vi "FPGA_Global.vi"() -> ()   [LabVIEW 2011]
panel:
  in  "Number of Modulation Points":u8
  in  "Cycles per Modulation":u32
  in  "Saturated Position Step":i32
  in  "Mobility Update?":bool
  in  "Cycles per Square Wave":u16
  in  "Square Voltage (y)":i16
  in  "Square Voltage (x)":i16
  in  "Inverse Mobility":i32
  in  "Inverse Diffusion Constant":u32
  in  "Sub-Bin Delay (ticks)":u16
  in  "Bins per Cycle":u8
  in  "Bin Period (ticks)":u16
  in  "Go":bool
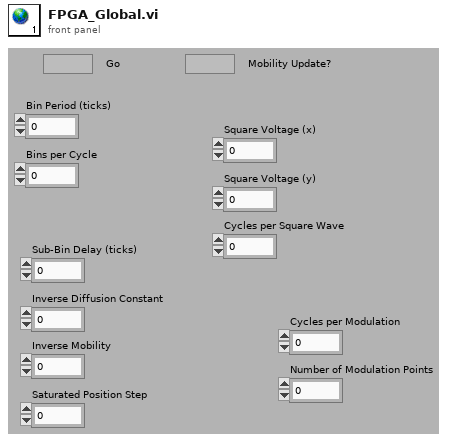
[diagram p1: front panel]
diagram:
